vi "Compteur_non_reentrant.vi"() -> (0 "Compteur":dbl)   [LabVIEW 2020]
doc: "Compteur 1"
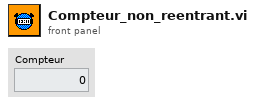
[diagram p1: front panel]
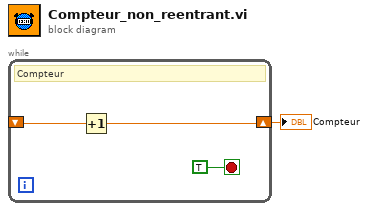
[diagram p0: block diagram]
diagram:
  n1 = while {
    shift-right: [w2] -> w1
    shift-left: _ -> [w3]
    stop <- TRUE stop-if-true
    # "Compteur"
    n2 = Increment(x=w3) -> (x+1=w2:dbl)
  }
  "Compteur" <- w1
